vi "Set Windows Position.vi"(7 "pos":T1, 8 "error in (no error)":errorcluster, 9 "uFlags":u32(ring)=1 items=["SWP_ASYNCWINDOWPOS"=16384, "SWP_DEFERERASE"=8192, "SWP_DRAWFRAME"=32, "SWP_HIDEWINDOW"=128, "SWP_NOACTIVATE"=16, "SWP_NOCOPYBITS"=256, "SWP_NOMOVE"=2, "SWP_NOOWNERZORDER"=512, "SWP_NOREDRAW"=8, "SWP_NOSENDCHANGING"=1024, "SWP_NOSIZE"=1, "SWP_NOZORDER"=4, "SWP_SHOWWINDOW"=64], 10 "hWndInsertAfter":string(combo), 11 "hWnd":u32) -> (0 "error out":errorcluster, 3 "hWnd out":u32)   [LabVIEW 2025]
uses:
  user32.dll
  Test Unit.lvlib
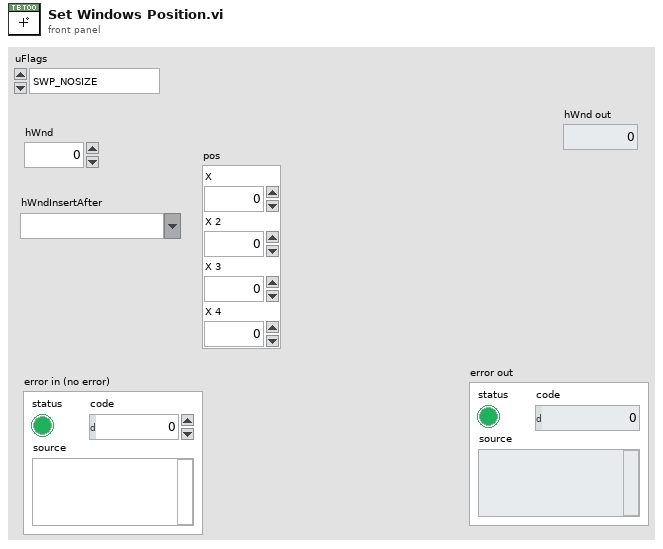
[diagram p1: front panel]
types:
  T1 = cluster{"X":i32, "X 2":i32, "X 3":i32, "X 4":i32}
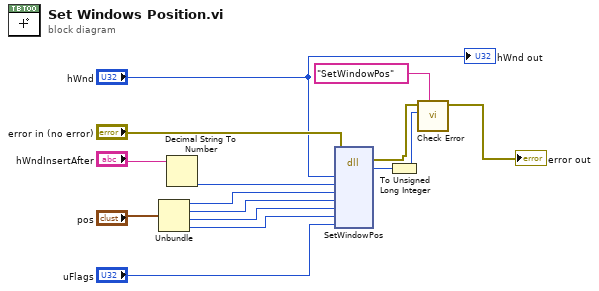
[diagram p0: block diagram]
diagram:
  n1 = Unbundle("pos") -> ("X"=w14:i32, "X 2"=w13:i32, "X 3"=w12:i32, "X 4"=w11:i32)
  n2 = Decimal String To Number(string="hWndInsertAfter") -> (number=w9:i32)  [unwired: 2 in, 1 out]
  n3 = dll-call lib="USER32.DLL" fn="SetWindowPos"(error in="error in (no error)", "hWnd"="hWnd", "hWndInsertAfter"=w9, "left"=w14, "top"=w13, "width"=w12, "height"=w11, "fuFlags"="uFlags") -> (error out=w6:errorcluster, "error"=w4:i32)  [unwired: 9 in, 1 out]
  n4 = To Unsigned Long Integer(number=w4) -> (unsigned 32bit integer=w2:u32)
  n5 = call "Check Error.vi"("Description"="SetWindowPos", "Return Code"=w2, "error in (no error)"=w6) -> ("error out"=→"error out":errorcluster)  [unwired: 8 in]
  "hWnd out" <- "hWnd"
